vi "Batch_convert_TDMS_format_folder.vi"() -> ()   [LabVIEW 2013]
panel:
  out "Current file":string
  in  "Folder to be converted":path
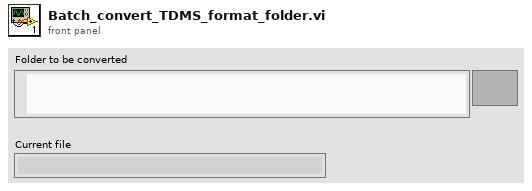
[diagram p1: front panel]
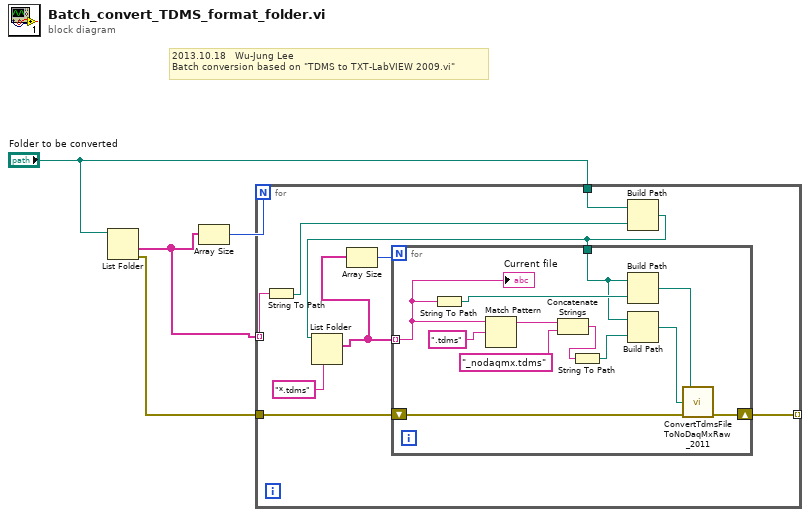
[diagram p0: block diagram]
diagram:
  # "2013.10.18   Wu-Jung Lee\nBatch conversion based on \"TDMS to TXT-LabVIEW 2009.vi\""
  n1 = List Folder(path="Folder to be converted") -> (folder names=w2:string[], error out=w4:errorcluster)  [unwired: 3 in, 2 out]
  n2 = Array Size(array=w2) -> (size(s)=w1:i32)
  n3 = for {
    N: w1 -> [_]
    tunnel: w4 -> [w12]
    tunnel: [w11] -> _ mode=indexing
    tunnel: "Folder to be converted" -> [w7]
    tunnel: w2 -> [w10] mode=indexing
    n4 = String To Path(string=w10) -> (path=w6:path)
    n5 = Build Path(base path=w7, name or relative path=w6) -> (appended path=w5:path)
    n6 = List Folder(path=w5, pattern="*.tdms") -> (filenames=w9:string[])  [unwired: 2 in, 3 out]
    n7 = Array Size(array=w9) -> (size(s)=w13:i32)
    n8 = for {
      N: w13 -> [_]
      tunnel: w9 -> [w25] mode=indexing
      shift-right: [w17] -> w11
      shift-left: w12 -> [w16]
      tunnel: w5 -> [w19]
      n9 = String To Path(string=w25) -> (path=w20:path)
      n10 = Match Pattern(string=w25, regular expression=".tdms") -> (before substring=w22:string)  [unwired: 1 in, 3 out]
      n11 = Concatenate Strings(w22, "_nodaqmx.tdms" ("string")) -> (w23:string)
      n12 = String To Path(string=w23) -> (path=w18:path)
      n13 = Build Path(base path=w19, name or relative path=w20) -> (appended path=w14:path)
      n14 = Build Path(base path=w19, name or relative path=w18) -> (appended path=w15:path)
      n15 = call "ConvertTdmsFileToNoDaqMxRaw_2011.vi"("Error In"=w16, "File conver to"=w15, "File convert from"=w14) -> ("Error Out"=w17:errorcluster)  [unwired: 5 in]
      "Current file" <- w25
    }
  }
